vi "挥发酚启动命令.vi"(8 "error in (no error)":errorcluster, 11 "参数":T1={"站号"=1, "量程切换"=enum."AUTO", "控制命令"=enum."启动测量", "模式设置"=enum."待机", "测量间隔"=0} {"站号" items=["总磷"=1, "总氮"=2, "氨氮"=3, "CODMn"=21]}) -> (0 "error out":errorcluster)   [LabVIEW 2016, in "质控单元V4.lvlib"]
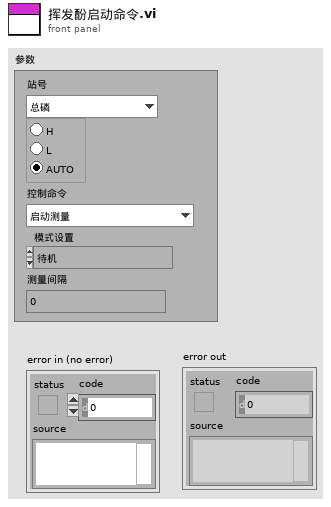
[diagram p1: front panel]
types:
  T1 = cluster{"站号":u16, "量程切换":enum32{"H", "L", "AUTO"}, "控制命令":enum16{"启动测量", "标样核查", "零点核查", "跨度核查", "空白测试", "平行样测试", "加标回收", "空白校准", "标样校准", "初始化（清洗）", "停止测试", "仪器重启", "校时", "模式设置", "测量间隔设置"}, "模式设置":enum16{"待机", "连续模式", "周期模式", "定点模式", "受控模式", "手动模式"}, "测量间隔":u16}
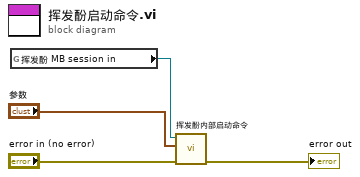
[diagram p0: block diagram]
diagram:
  n1 = global read "系统交互.vi" "挥发酚 MB session in"() -> (w1:refnum<class "MB_Master.lvclass">)
  n2 = call "挥发酚内部启动命令.vi"("error in (no error)"="error in (no error)", "参数"="参数", "MB session in"=w1) -> ("error out"=→"error out":errorcluster)  [unwired: 8 in]
